vi "DepthProfileWriteCore.vi"(7 "Buffer In":T1(array[cluster]), 8 "error in":errorcluster, 9 "RepRate (Hz)":dbl=500.0, 10 "Total_Depth (shots)":i32=500, 11 "pre-Processed_Buffer":refnum<queue>) -> (0 "error out":errorcluster, 5 "Buffer Out":T1(array[cluster]))   [LabVIEW 2012]
panel:
  out "# elements in queue":i32
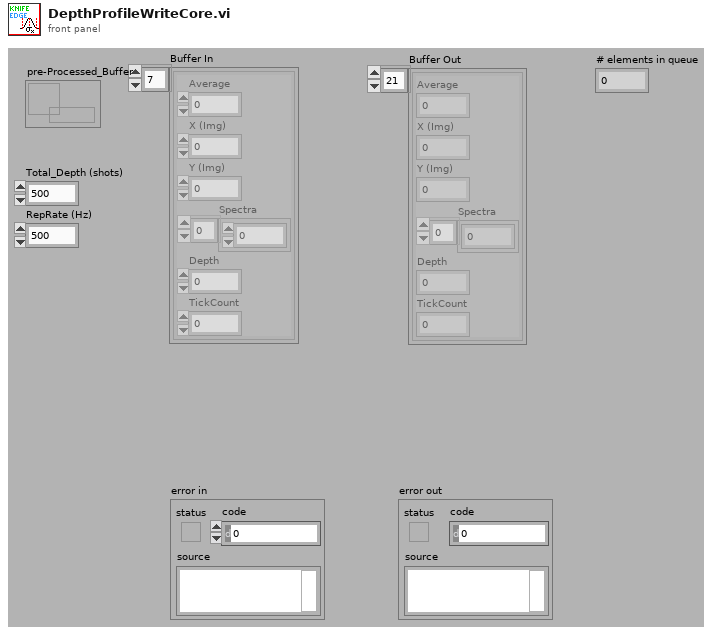
[diagram p1: front panel]
types:
  T1 = cluster{"Average":i32, "X (Img)":i32, "Y (Img)":i32, "Spectra":sgl[], "Depth":i32, "TickCount":dbl}[]
  T2 = cluster{"Average":i32, "X (Img)":i32, "Y (Img)":i32, "Spectra":sgl[], "Depth":i32, "TickCount":dbl}
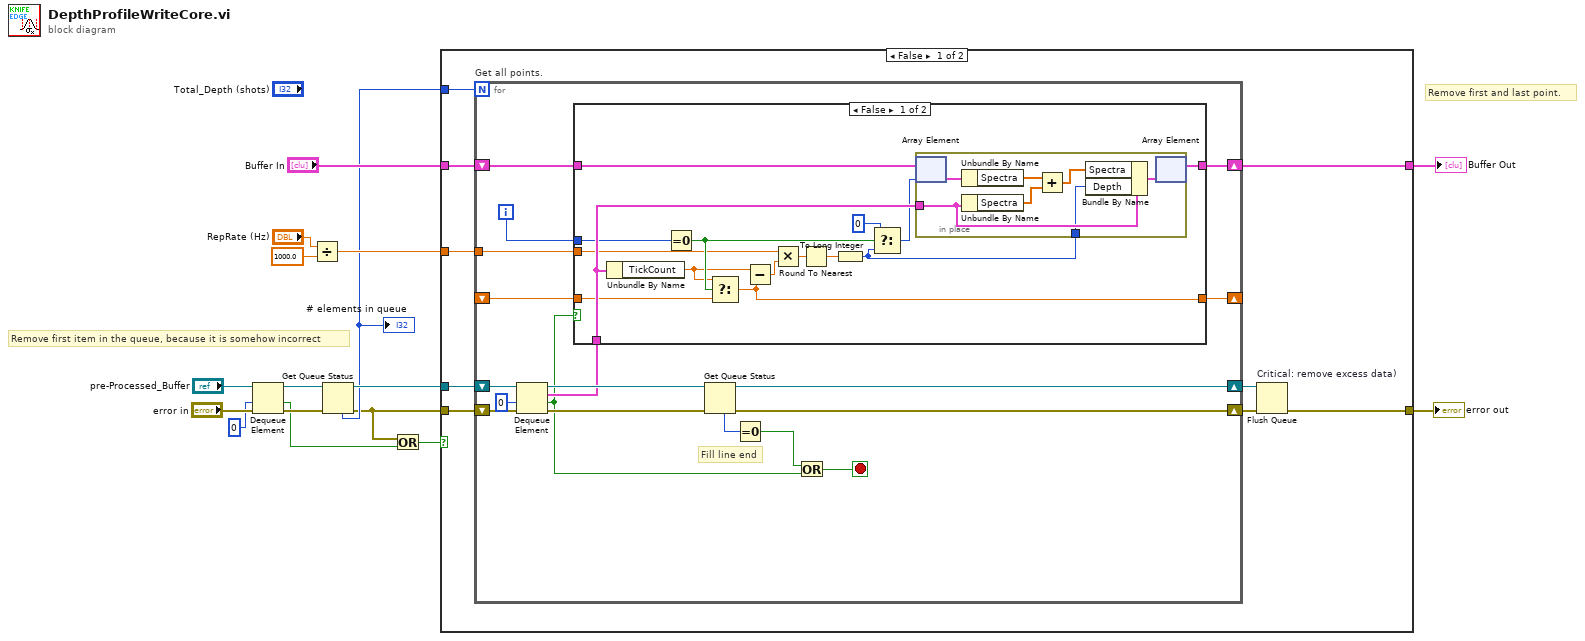
[diagram p0: block diagram]
diagram:
  # "Remove first item in the queue, because it is somehow incorrect"
  # "Remove first and last point."
  n1 = Dequeue Element ("Somehow, the first item is empty not real signal.")(queue="pre-Processed_Buffer", timeout in ms (-1)=0, error in (no error)="error in") -> (queue out=w12:refnum<queue>, timed out?=w1:bool, error out=w6:errorcluster)  [unwired: 1 out]
  n2 = Divide(x="RepRate (Hz)", y=1000.0 ("x")) -> (x/y=w14:dbl)
  n3 = Get Queue Status(queue=w12, error in (no error)=w6) -> (queue out=w7:refnum<queue>, error out=w2:errorcluster, # elements in queue=w5:i32)  [unwired: 1 in, 5 out]
  "# elements in queue" <- w5
  n4 = Or(x=w2, y=w1) -> (x .or. y?=w3:bool)
  n5 = case shown="False" w3 {
    tunnel: [w21 w67] -> w16
    tunnel: w7 -> [w18 _]
    tunnel: w5 -> [w25 _]
    tunnel: w14 -> [w24 _]
    tunnel: "Buffer In" -> [w20 w68]
    tunnel: [w19 w68] -> w8
    tunnel: w2 -> [w17 w67]
    frame False {
      n6 = for "Get all points." {
        N: w25 -> [_]
        shift-right: [w40] -> w23
        shift-left: w17 -> [w42]
        shift-right: [w36] -> w19
        shift-left: w20 -> [w37]
        shift-right: [w30] -> _
        shift-left: _ -> [w32]
        tunnel: w24 -> [w31]
        shift-right: [w29] -> w22
        shift-left: w18 -> [w41]
        i -> [w33]
        stop <- w27 stop-if-true
        # "Fill line end"
        n7 = Dequeue Element(queue=w41, timeout in ms (-1)=0, error in (no error)=w42) -> (queue out=w39:refnum<queue>, element=w34:T2, timed out?=w26:bool, error out=w40:errorcluster)
        n8 = case shown="False" w26 {
          tunnel: w37 -> [w57 w66]
          tunnel: [w56 w66] -> w36
          tunnel: w34 -> [w55 _]
          tunnel: w33 -> [w54 _]
          tunnel: w32 -> [w51 w65]
          tunnel: w31 -> [w48 _]
          tunnel: [w46 w65] -> w30
          frame False {
            n9 = Unbundle By Name(w55) -> ("TickCount"=w50:dbl)
            n10 = Equal To 0?(x=w54) -> (x = 0?=w53:bool)
            n11 = Select(t=w50, s=w53, f=w51) -> (s? t:f=w46:dbl)
            n12 = Subtract(x=w50, y=w46) -> (x-y=w44:dbl)
            n13 = Multiply(x=w48, y=w44) -> (x*y=w49:dbl)
            n14 = Round To Nearest(number=w49) -> (nearest integer value=w47:dbl)
            n15 = To Long Integer(number=w47) -> (32bit integer=w43:i32)
            n16 = Select(t=0, s=w53, f=w43) -> (s? t:f=w45:i32)
            n17 = in-place {
              in-place-border: w55 -> [w60]
              in-place-border: w43 -> [w58]
              n18 = in-place-array #1(w57, w45) -> (w64:T2)
              n19 = Unbundle By Name(w64) -> ("Spectra"=w63:sgl[])
              n20 = Unbundle By Name(w60) -> ("Spectra"=w62:sgl[])
              n21 = Add(x=w63, y=w62) -> (x+y=w59:sgl[])
              n22 = Bundle By Name(cluster=w60, "Spectra"=w59, "Depth"=w58) -> (w61:T2)
              n23 = in-place-array #1(w61) -> (w56:T1)  [unwired: 1 out]
            }
          }
          frame True {
          }
        }
        n24 = Get Queue Status(queue=w39) -> (queue out=w29:refnum<queue>, # elements in queue=w38:i32)  [unwired: 2 in, 6 out]
        n25 = Equal To 0?(x=w38) -> (x = 0?=w35:bool)
        n26 = Or(x=w35, y=w26) -> (x .or. y?=w27:bool)
      }
      n27 = Flush Queue "Critical: remove excess data)"(queue=w22, error in (no error)=w23) -> (error out=w21:errorcluster)  [unwired: 2 out]
    }
    frame True {
    }
  }
  "error out" <- w16
  "Buffer Out" <- w8
